vi "libssh2_sftp_statvfs.vi"(8 "error in (no error)":errorcluster, 10 "path":string, 11 "sftp":T2) -> (0 "error out":errorcluster, 2 "statvfs":T1)   [LabVIEW 2013, in "libssh2.lvlib"]
doc: "Get file system statistics."
uses:
  libssh2.lvlib
  SFTP Refnum.ctl
  libssh2_sftp_statvfs.ctl
  Not a SFTP Refnum.vi
  <vilib>/Utility/error.llb/Error Cluster From Error Code.vi
  Global Settings.vi
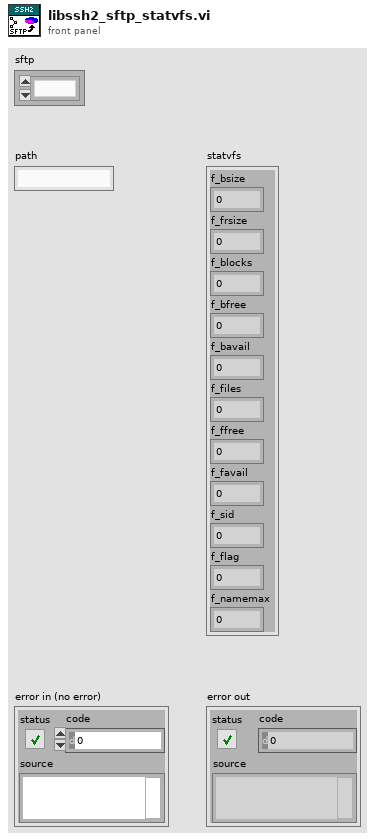
[diagram p1: front panel]
types:
  T1 = typedef "libssh2.lvlib/libssh2_sftp_statvfs.ctl" = cluster{"f_bsize":u64, "f_frsize":u64, "f_blocks":u64, "f_bfree":u64, "f_bavail":u64, "f_files":u64, "f_ffree":u64, "f_favail":u64, "f_sid":u64, "f_flag":u64, "f_namemax":u64}
  T2 = typedef "libssh2.lvlib/SFTP Refnum.ctl" = refnum<k1>
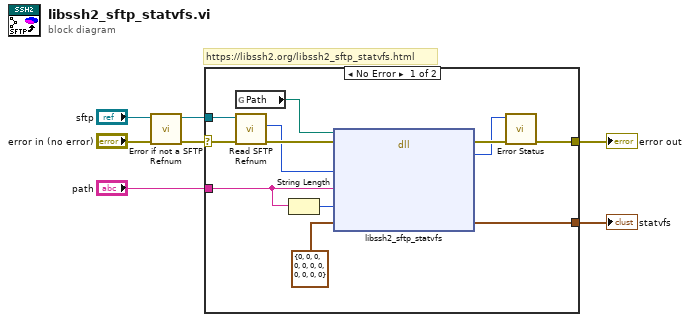
[diagram p0: block diagram]
diagram:
  # "https://libssh2.org/libssh2_sftp_statvfs.html"
  n1 = call "Error if not a SFTP Refnum.vi"("error in (no error)"="error in (no error)", "sftp"="sftp") -> ("error out"=w6:errorcluster, "sftp out"=w5:T2)  [unwired: 8 in]
  n2 = case shown="No Error" w6 {
    selector: w6 -> [w18 w20]
    tunnel: w5 -> [w17 _]
    tunnel: [w13 w20] -> w4
    tunnel: "path" -> [w10 _]
    tunnel: [w8 _] -> w1
    frame No Error {
      n3 = global read "Global Settings.vi" "Path"() -> (w19:path)
      n4 = call "Read SFTP Refnum.vi"("error in (no error)"=w18, "sftp"=w17) -> ("error out"=w16:errorcluster, "LIBSSH2_SFTP*"=w15:u64)  [unwired: 8 in]
      n5 = String Length(string=w10) -> (length=w11:i32)
      n6 = dll-call lib="?" fn="libssh2_sftp_statvfs"(path in=w19, error in=w16, "sftp"=w15, "path"=w10, "path_len"=w11, "st"=T1 {"f_bsize"=0, "f_frsize"=0, "f_blocks"=0, "f_bfree"=0, "f_bavail"=0, "f_files"=0, "f_ffree"=0, "f_favail"=0, "f_sid"=0, "f_flag"=0, "f_namemax"=0} ("statvfs")) -> (error out=w14:errorcluster, "return value"=w12:i32, "st"=w8:T1)  [unwired: 4 in, 1 out]
      n7 = call "Error Status.vi"("error in (no error)"=w14, "return value"=w12) -> ("error out"=w13:errorcluster)  [unwired: 8 in, 1 out]
    }
    frame Error {
    }
  }
  "error out" <- w4
  "statvfs" <- w1
